vi "New Message Command (BC-RT).vi"(6 "monitor (F)":bool, 8 "error in":errorcluster, 9 "Message Command Configuration":T1, 10 "messageBufferIDRef":i32, 11 "name":string) -> (0 "error out":errorcluster, 2 "Message Command ID out":i32, 3 "new message command":refnum<k24>)   [LabVIEW 2020, in "Ballard_1553_Hardware_ni.lvlib"]
uses:
  Ballard_1553_Hardware_ni.lvlib
  C:/Users/Administrator/Desktop/GIT/Ballard-MIL-STD-1553-Custom-Device/Source/System Explorer/SubVIs/Parse XML Ballard/1.2/BTIXML_SerDes.dll
  Ballard-MIL-STD-1553-Custom-Device/Source/System Explorer/SubVIs/Parse XML Ballard/1.2/BTIXML_SerDes.dll
  _typedefs/MessageCommand_BCRT_type.ctl
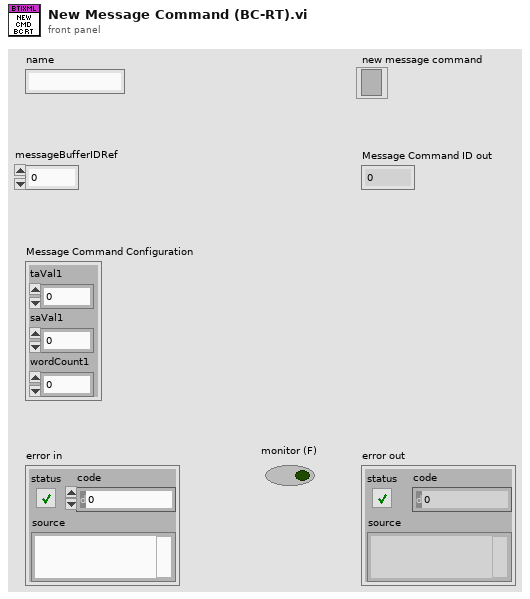
[diagram p1: front panel]
types:
  T1 = typedef "Ballard_1553_Hardware_ni.lvlib/MessageCommand_BCRT_type.ctl" = cluster{"taVal1":i8, "saVal1":i8, "wordCount1":i8}
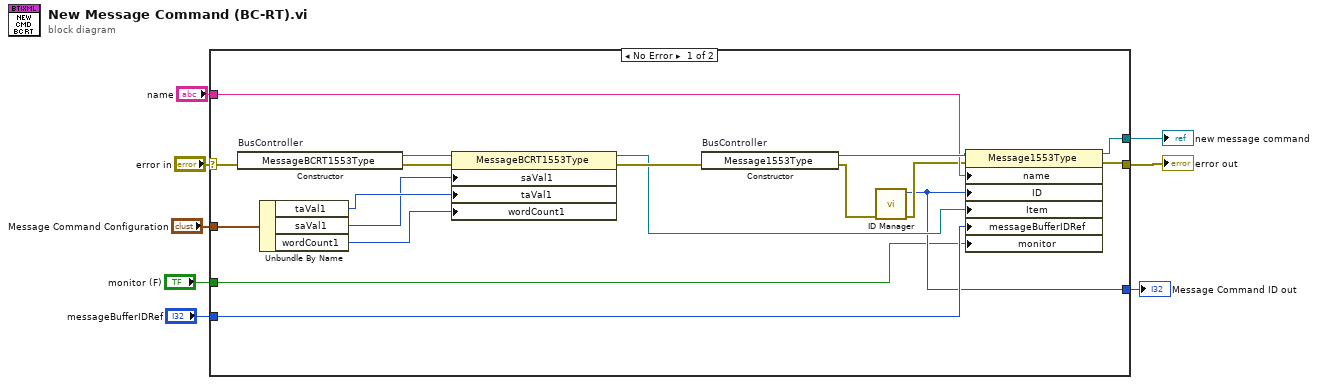
[diagram p0: block diagram]
diagram:
  n1 = case shown="No Error" "error in" {
    selector: "error in" -> [w26 w27]
    tunnel: [w17 w27] -> w7
    tunnel: "name" -> [w20 _]
    tunnel: "messageBufferIDRef" -> [w18 _]
    tunnel: [w16 _] -> w4
    tunnel: "Message Command Configuration" -> [w15 _]
    tunnel: [w10 _] -> w2
    tunnel: "monitor (F)" -> [w9 _]
    frame No Error {
      n2 = constructor on="BusController" class="MessageBCRT1553Type"(error in=w26) -> (reference out=w25:refnum<k24>, error out=w24:errorcluster)  [unwired: 2 in, 1 out]
      n3 = Unbundle By Name(w15) -> ("taVal1"=w14:i8, "saVal1"=w13:i8, "wordCount1"=w12:i8)
      n4 = property class="MessageBCRT1553Type"(reference=w25, error in=w24, "saVal1"=w13, "taVal1"=w14, "wordCount1"=w12) -> (reference out=w11:refnum<k24>, error out=w22:errorcluster)
      n5 = constructor on="BusController" class="Message1553Type"(error in=w22) -> (reference out=w23:refnum<k24>, error out=w21:errorcluster)  [unwired: 2 in, 1 out]
      n6 = call "ID Manager.vi"("error in"=w21) -> ("error out"=w19:errorcluster, "ID out"=w10:i32)  [unwired: 9 in]
      n7 = property class="Message1553Type"(reference=w23, error in=w19, "name"=w20, "ID"=w10, "Item"=w11, "messageBufferIDRef"=w18, "monitor"=w9) -> (reference out=w16:refnum<k24>, error out=w17:errorcluster)
    }
    frame Error {
    }
  }
  "error out" <- w7
  "new message command" <- w4
  "Message Command ID out" <- w2
